vi "VCS Restore.vi"(8 "error in (no error)":errorcluster, 11 "axis in":cluster{"keyHandle":u32, "nodeId":u16}={"keyHandle"=0, "nodeId"=1}) -> (0 "error out":errorcluster, 3 "axis out":cluster{"keyHandle":u32, "nodeId":u16}={"keyHandle"=0, "nodeId"=1})   [LabVIEW 2010]
doc: "<B>VCS Restore</B> restores all default parameters."
uses:
  Resources/EposCmd.dll
  Resources/EposCmd64.dll
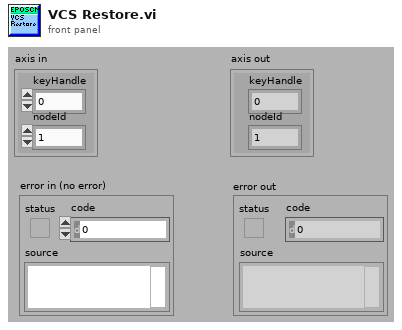
[diagram p1: front panel]
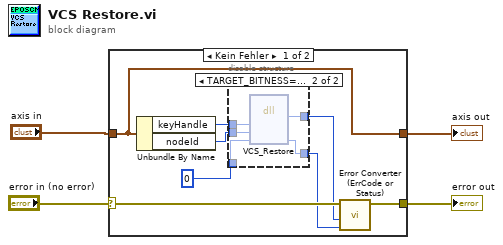
[diagram p0: block diagram]
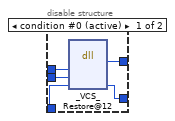
[diagram p2: hidden frame]
diagram:
  n1 = case shown="Kein Fehler" "error in (no error)" {
    selector: "error in (no error)" -> [w11 w24]
    tunnel: [w10 w24] -> w3
    tunnel: "axis in" -> [w6 w23]
    tunnel: [w6 w23] -> w1
    frame No Error {
      n2 = Unbundle By Name(w6) -> ("keyHandle"=w8:u32, "nodeId"=w7:u16)
      n3 = disable-structure shown="TARGET_BITNESS==64" {
        disable-tunnel: u32 0 ("pErrorCode") -> [w17 w22]
        disable-tunnel: [w16 w21] -> w9
        disable-tunnel: w8 -> [w15 w20]
        disable-tunnel: w7 -> [w14 w19]
        disable-tunnel: [w13 w18] -> w5
        frame condition #0 (active) {
          n4 = dll-call lib="C:/Sources/LabView/maxon EPOS/Resources/EposCmd.*" fn="_VCS_Restore@12"("KeyHandle"=w15, "NodeId"=w14, "pErrorCode"=w17) -> (w13:i32, "pErrorCode"=w16:u32)  [unwired: 5 in, 2 out]
        }
        frame condition #1 {
          n5 = dll-call lib="C:/setup/Resources/EposCmd64.*" fn="VCS_Restore" ("EposCmd.dll:_VCS_Restore@12")("KeyHandle"=w20, "NodeId"=w19, "pErrorCode"=w22) -> ("Rückgabetyp"=w18:i32, "pErrorCode"=w21:u32)  [unwired: 5 in, 2 out]
        }
      }
      n6 = call "Error Converter (ErrCode or Status).vi"("error code"=w9, "return type"=w5, "error in (no error)"=w11) -> ("error out"=w10:errorcluster)  [unwired: 7 in]
    }
    frame Error {
    }
  }
  "error out" <- w3
  "axis out" <- w1
